vi "Plotmatrix Appearance Page.vi"() -> ()   [LabVIEW 2020, in "XY Plot Matrix.lvclass"]
uses:
  <vilib>/Math Plots/2D Math Plots/XY Plot Matrix/XY Plot Matrix/XY Plot Matrix.lvclass
  <vilib>/Math Plots/2D Math Plots/2D Plot/2D Plot/Typedef/Graph General Property.ctl
  <vilib>/Math Plots/2D Math Plots/2D Plot/Action String/XYPlotMatrix Ctrl Act Queue.ctl
  <vilib>/Math Plots/2D Math Plots/2D Plot/Action String/XYPlotMatrix Ctrl Act Cluster.ctl
  <vilib>/Math Plots/2D Math Plots/2D Plot/Action String/2DMathPlot State Class.ctl
  <vilib>/Math Plots/2D Math Plots/2D Plot/2D Plot/Typedef/Dialog State.ctl
  <vilib>/Math Plots/2D Math Plots/2D Plot/2D Plot/Typedef/Temp Graph Property Action.ctl
  <vilib>/Math Plots/2D Math Plots/2D Plot/2D Plot/Typedef/Temp Graph State.ctl
  <vilib>/Math Plots/2D Math Plots/2D Plot/2D Plot/2D Plot.lvclass
panel:
  in  "Event Registration":refnum<event-registration>
  in  "Control Ref Queue":T1
  out "Graph General Out":T2
  in  "Graph General In":T2
  in  "Legend:Plots Shown":u32=1 caption="Plots shown" min=1
  in  "Autosize Legend":bool caption="Auto size to plot names"
  in  "Legend:Visible":bool caption="Show plot legend"
  in  "Palette:Visible":bool caption="Show graph palette"
  in  "Height":u32 step=1
  in  "Width":u32 step=1
  in  "Enabled State":T3(radio)
  in  "Caption.Visible":bool caption="Caption"
  in  "Caption.Text":string caption="Caption Text"
  in  "Label.Text":string caption="Label Text"
  in  "Label.Visible":bool caption="Label"
  # "Caption"
  # "Label"
  # "Enabled State"
  # "Size"
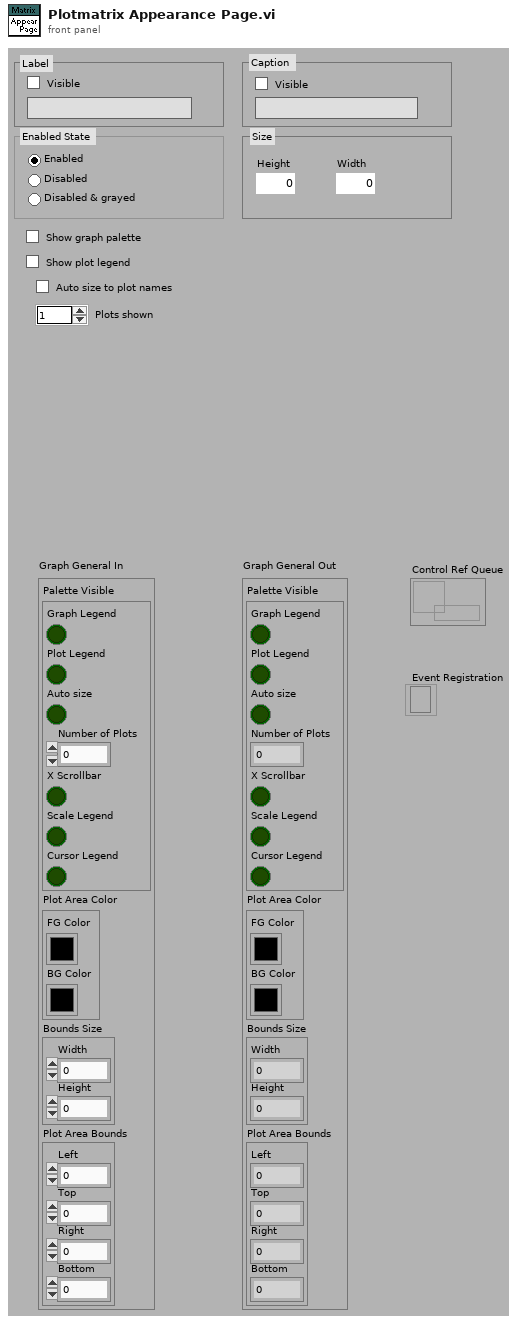
[diagram p1: front panel]
types:
  T1 = typedef "XYPlotMatrix Ctrl Act Queue.ctl" = refnum<queue>
  T2 = typedef "2D Plot.lvclass/Graph General Property.ctl" = cluster{"Palette Visible":cluster{"Graph Legend":bool, "Plot Legend":bool, "Auto size":bool, "Number of Plots":u32, "X Scrollbar":bool, "Scale Legend":bool, "Cursor Legend":bool}, "Plot Area Color":cluster{"FG Color":u32, "BG Color":u32}, "Bounds Size":cluster{"Width":u32, "Height":u32}, "Plot Area Bounds":cluster{"Left":i16, "Top":i16, "Right":i16, "Bottom":i16}}
  T3 = enum32{"Enabled", "Disabled", "Disabled & grayed", "Multiple Values"}
  T4 = typedef "2D Plot.lvclass/Dialog State.ctl" = enum16{"Initialize", "Read Property", "Write Property", "Idle", "Exit"}
  T5 = typedef "XYPlotMatrix Ctrl Act Cluster.ctl" = cluster{"Facade VI":refnum<vi>, "XControl":refnum<vi>, "Sub Panel":refnum<vi>, "Sub VI":refnum<vi>, "Export Image":refnum<vi>, "Display State Change Class":T6}
  T6 = typedef "2DMathPlot State Class.ctl" = enum16{"Update All (Undo)", "Update General", "Update Appearance", "Update Format", "Update Scale", "Update Marker", "Update Cursor", "None"}
  T7 = typedef "2D Plot.lvclass/Temp Graph State.ctl" = enum16{"Create", "Update Graph", "Update Property Only", "Get Plot Name", "Get Axis Name", "Destory"}
  T8 = typedef "2D Plot.lvclass/Temp Graph Property Action.ctl" = enum16{"Appearance Property", "Format Property", "Plots Property", "Scales Property"}
  T9 = enum8{"Enabled", "Disabled", "Disabled and Grayed Out"}
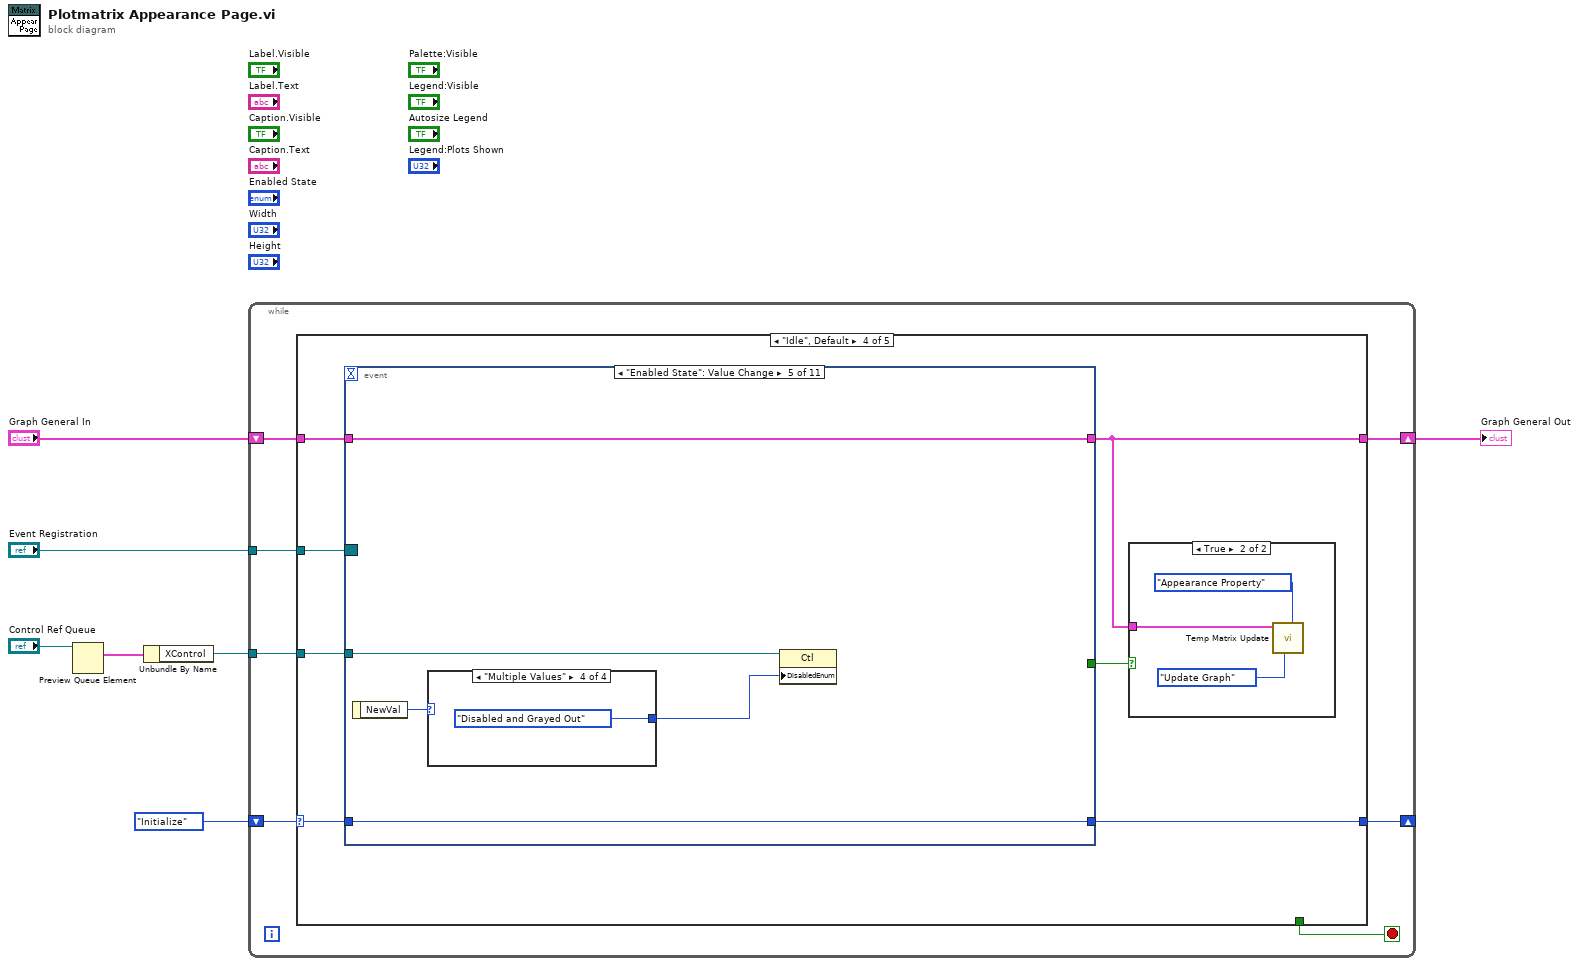
[diagram p0: block diagram]
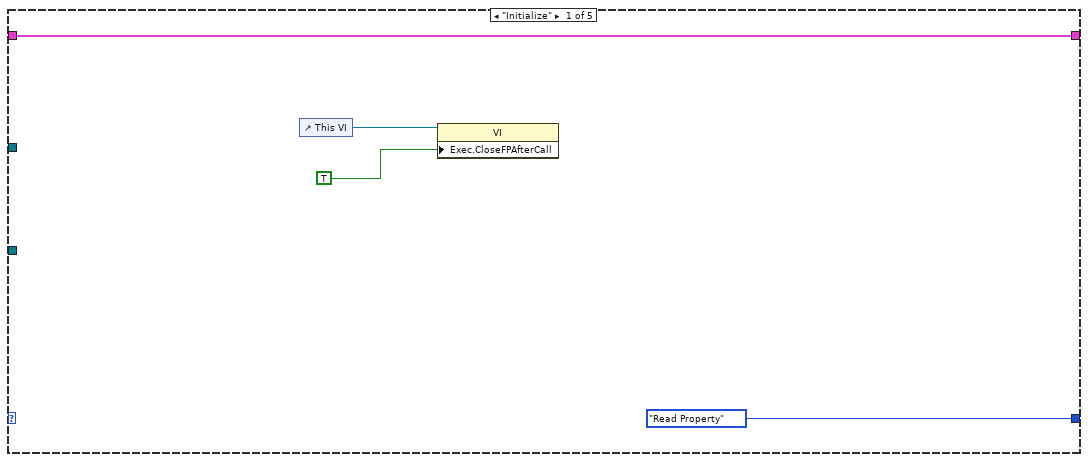
[diagram p2: hidden frame]
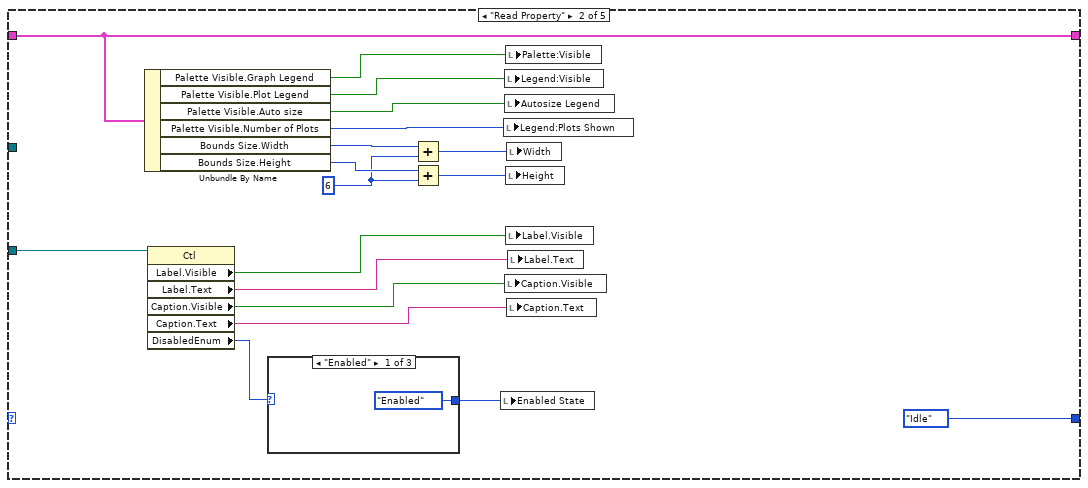
[diagram p3: hidden frame]
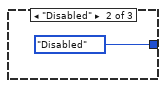
[diagram p4: hidden frame]
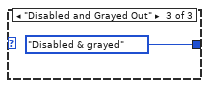
[diagram p5: hidden frame]
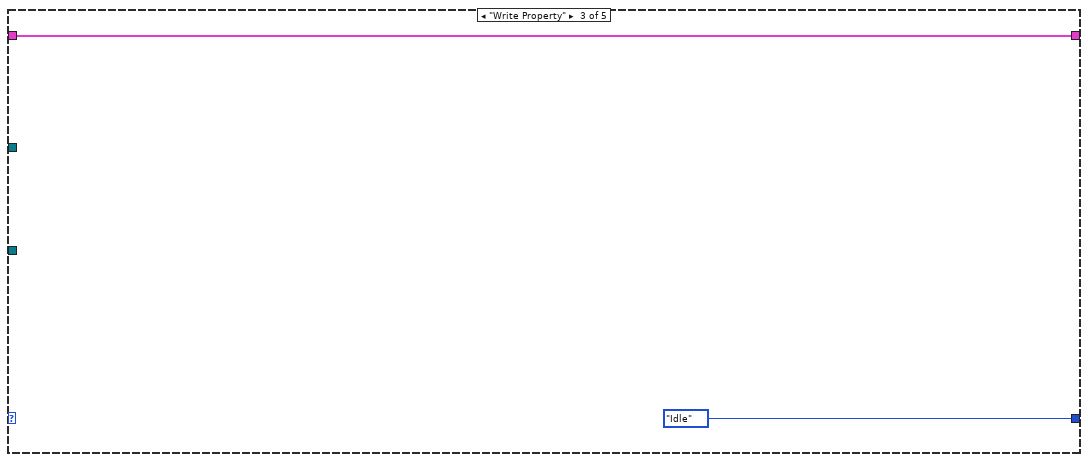
[diagram p6: hidden frame]
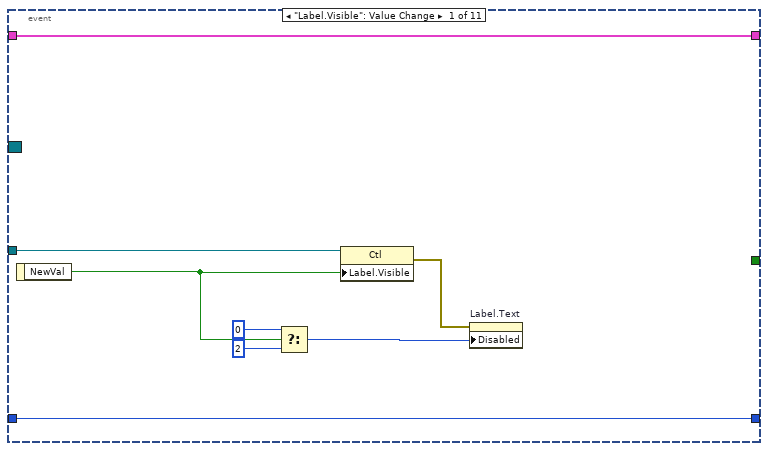
[diagram p8: hidden frame]
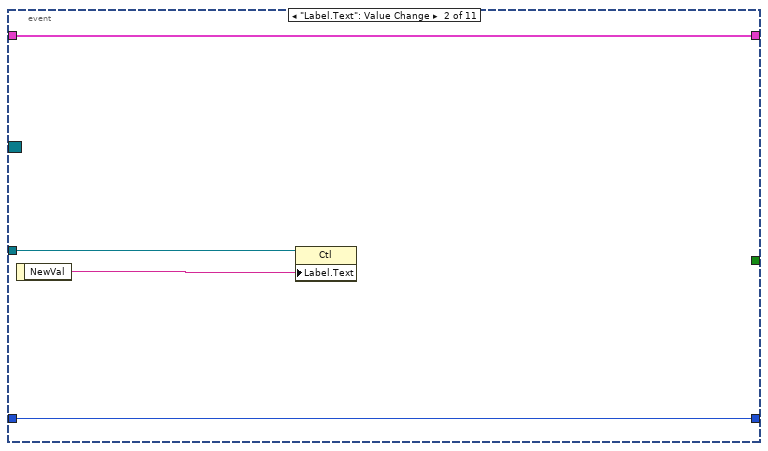
[diagram p9: hidden frame]
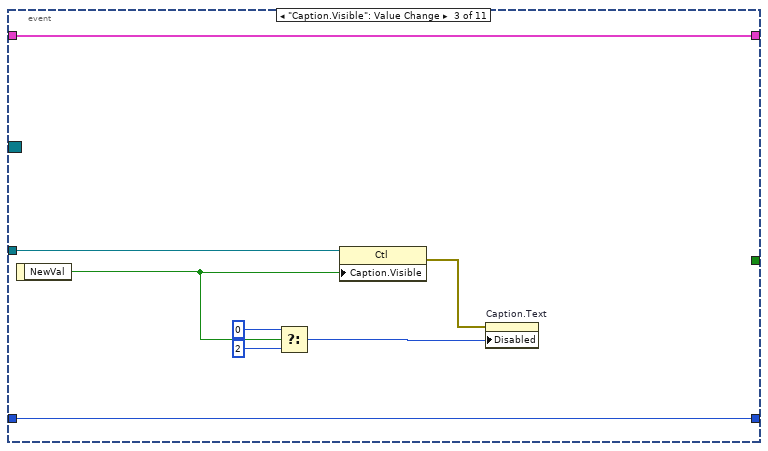
[diagram p10: hidden frame]
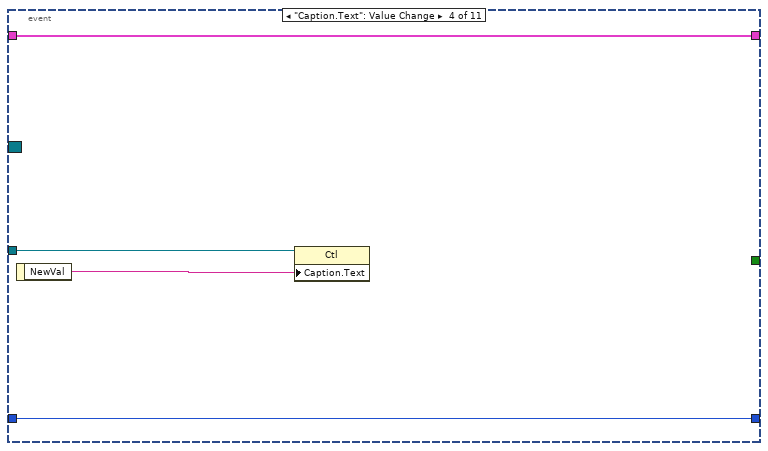
[diagram p11: hidden frame]
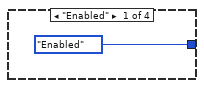
[diagram p12: hidden frame]
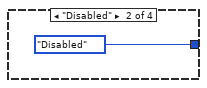
[diagram p13: hidden frame]
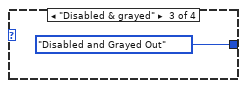
[diagram p14: hidden frame]
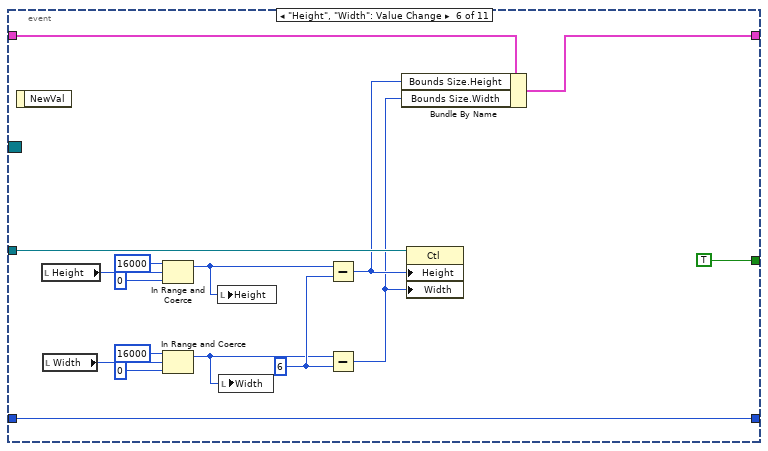
[diagram p15: hidden frame]
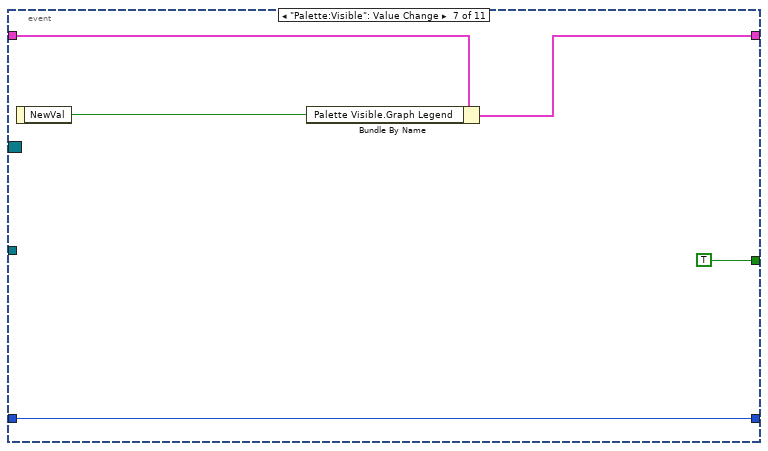
[diagram p16: hidden frame]
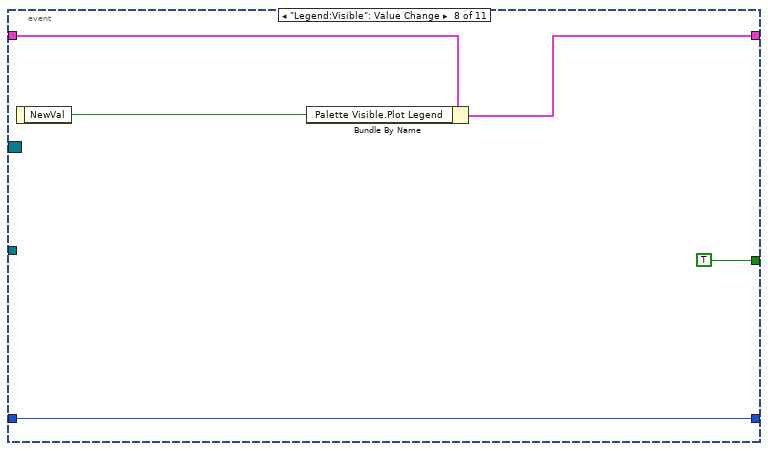
[diagram p17: hidden frame]
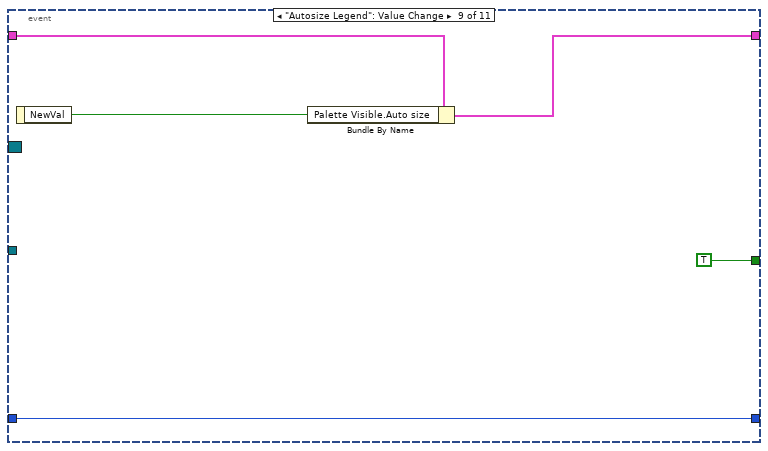
[diagram p18: hidden frame]
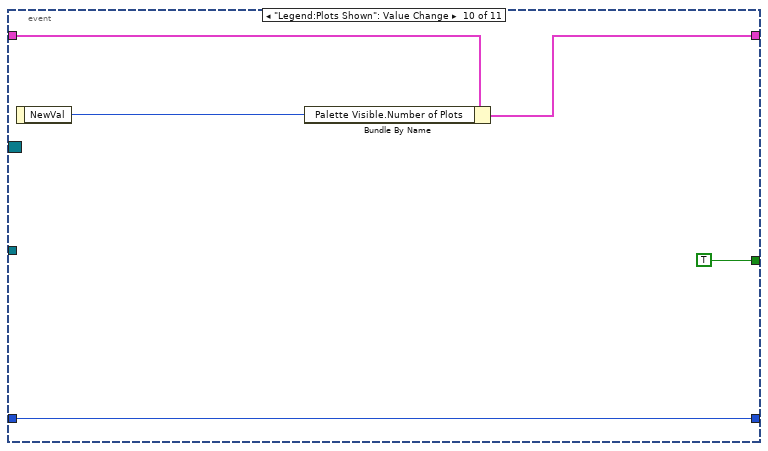
[diagram p19: hidden frame]
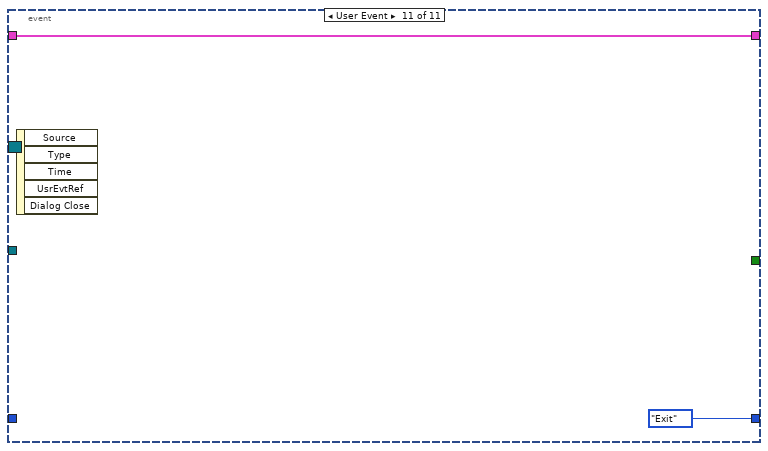
[diagram p20: hidden frame]
diagram:
  n1 = Preview Queue Element(queue="Control Ref Queue") -> (element=w1:T5)  [unwired: 1 in, 4 out]
  n2 = Unbundle By Name(w1) -> ("XControl"=w3:refnum<vi>)
  n3 = while {
    shift-right: [w12] -> _
    shift-left: Dialog_State."Initialize" ("Enum") -> [w14]
    shift-right: [w11] -> w6
    shift-left: "Graph General In" -> [w10]
    tunnel: w3 -> [w9]
    tunnel: "Event Registration" -> [w8]
    stop <- w13 stop-if-true
    n4 = case shown="\"Idle\", Default" w14 {
      selector: w14 -> [_ _ _ w44 w124]
      tunnel: [_ _ _ _ TRUE] -> w13
      tunnel: [Dialog_State."Read Property" ("Enum") Dialog_State."Idle" ("Enum") Dialog_State."Idle" ("Enum") w45 w124] -> w12
      tunnel: [w15 w26 w40 w42 w123] -> w11
      tunnel: w10 -> [w15 w26 w40 w48 w123]
      tunnel: w9 -> [_ w31 _ w47 _]
      tunnel: w8 -> [_ _ _ w46 _]
      frame "Initialize" {
        n5 = control-ref of="This VI"() -> (w17:refnum<vi>)
        n6 = property class="VI"(reference=w17, "Exec.CloseFPAfterCall"=TRUE ("Execution:Close After Call")) -> ()  [unwired: 1 in, 2 out]
      }
      frame "Read Property" {
        w21 = u32 6 ("y")
        n7 = Unbundle By Name(w26) -> ("Palette Visible.Graph Legend"=w35:bool, "Palette Visible.Plot Legend"=w34:bool, "Palette Visible.Auto size"=w33:bool, "Palette Visible.Number of Plots"=w32:u32, "Bounds Size.Width"=w25:u32, "Bounds Size.Height"=w24:u32)
        n8 = property class="Ctl"(reference=w31) -> ("Label.Visible"=w30:bool, "Label.Text"=w29:string, "Caption.Visible"=w28:bool, "Caption.Text"=w27:string, "DisabledEnum"=w20:T9)  [unwired: 1 in, 2 out]
        n9 = case shown="\"Enabled\"" w20 {
          tunnel: [T3."Enabled" ("Enabled State") T3."Disabled" ("Enabled State") T3."Disabled & grayed" ("Enabled State")] -> w19
          frame "Enabled" {
          }
          frame "Disabled" {
          }
          frame "Disabled and Grayed Out" {
          }
        }
        n10 = Add(x=w25, y=w21) -> (x+y=w23:u32)
        n11 = Add(x=w24, y=w21) -> (x+y=w22:u32)
        n12 = local write "Enabled State"(w19) -> ()
        n13 = local write "Legend:Plots Shown"(w32) -> ()
        n14 = local write "Legend:Visible"(w34) -> ()
        n15 = local write "Autosize Legend"(w33) -> ()
        n16 = local write "Caption.Visible"(w28) -> ()
        n17 = local write "Palette:Visible"(w35) -> ()
        n18 = local write "Height"(w22) -> ()
        n19 = local write "Label.Visible"(w30) -> ()
        n20 = local write "Width"(w23) -> ()
        n21 = local write "Caption.Text"(w27) -> ()
        n22 = local write "Label.Text"(w29) -> ()
      }
      frame "Write Property" {
      }
      frame "Idle", Default {
        n23 = event shown="[4] \"Enabled State\": Value Change" {
          selector: w46 -> [_ _ _ _ _ _ _ _ _ _ _]
          dyn-events: _ -> [_ _ _ _ _ _ _ _ _ _ _]
          timeout: _ -> [_ _ _ _ _ _ _ _ _ _ _]
          tunnel: w48 -> [w59 w61 w71 w73 w79 w100 w105 w110 w115 w120 w122]
          tunnel: [w59 w61 w71 w73 w79 w98 w104 w109 w114 w119 w122] -> w42
          tunnel: w47 -> [w58 w63 w70 w75 w80 w96 _ _ _ _ _]
          tunnel: [w52 w60 w64 w72 w78 w99 w102 w107 w112 w117 Dialog_State."Exit" ("Enum")] -> w45
          tunnel: w44 -> [w52 w60 w64 w72 w78 w99 w102 w107 w112 w117 _]
          tunnel: [_ _ _ _ _ TRUE TRUE TRUE TRUE TRUE _] -> w43
          event "Label.Visible": Value Change {
            n24 = event-data() -> ("NewVal"=w57:bool)  [unwired: 1 out]
            n25 = Select(t=u8 0 ("Disabled"), s=w57, f=u8 2 ("Disabled")) -> (s? t:f=w54:u8)
            n26 = property class="Ctl"(reference=w58, "Label.Visible"=w57) -> (error out=w53:errorcluster)  [unwired: 1 in, 1 out]
            n27 = property on="Label.Text" class="Str"(error in=w53, "Disabled"=w54) -> ()  [unwired: 1 in, 2 out]
          }
          event "Label.Text": Value Change {
            n28 = event-data() -> ("NewVal"=w62:string)  [unwired: 1 out]
            n29 = property class="Ctl"(reference=w63, "Label.Text"=w62) -> ()  [unwired: 1 in, 2 out]
          }
          event "Caption.Visible": Value Change {
            n30 = event-data() -> ("NewVal"=w69:bool)  [unwired: 1 out]
            n31 = Select(t=u8 0 ("Disabled"), s=w69, f=u8 2 ("Disabled")) -> (s? t:f=w66:u8)
            n32 = property class="Ctl"(reference=w70, "Caption.Visible"=w69) -> (error out=w65:errorcluster)  [unwired: 1 in, 1 out]
            n33 = property on="Caption.Text" class="Str"(error in=w65, "Disabled"=w66) -> ()  [unwired: 1 in, 2 out]
          }
          event "Caption.Text": Value Change {
            n34 = event-data() -> ("NewVal"=w74:string)  [unwired: 1 out]
            n35 = property class="Ctl"(reference=w75, "Caption.Text"=w74) -> ()  [unwired: 1 in, 2 out]
          }
          event "Enabled State": Value Change {
            n36 = event-data() -> ("NewVal"=w77:T3)  [unwired: 1 out]
            n37 = case shown="\"Multiple Values\"" w77 {
              tunnel: [T9."Enabled" ("Disabled") T9."Disabled" ("Disabled") T9."Disabled and Grayed Out" ("Disabled") T9."Disabled and Grayed Out" ("Disabled")] -> w76
              frame "Enabled" {
              }
              frame "Disabled" {
              }
              frame "Disabled & grayed" {
              }
              frame "Multiple Values" {
              }
            }
            n38 = property class="Ctl"(reference=w80, "DisabledEnum"=w76) -> ()  [unwired: 1 in, 2 out]
          }
          event "Height", "Width": Value Change {
            w93 = u32 6 ("x")
            n39 = event-data() -> ()  [unwired: 2 out]
            n40 = local read "Height"() -> (w88:u32)
            n41 = local read "Width"() -> (w87:u32)
            n42 = In Range and Coerce(upper limit=u32 16000, x=w88, lower limit=u32 0) -> (coerced(x)=w85:u32)  [unwired: 1 out]
            n43 = In Range and Coerce(upper limit=u32 16000, x=w87, lower limit=u32 0) -> (coerced(x)=w86:u32)  [unwired: 1 out]
            n44 = local write "Height"(w85) -> ()
            n45 = local write "Width"(w86) -> ()
            n46 = Subtract(x=w85, y=w93) -> (x-y=w95:u32)
            n47 = Subtract(x=w86, y=w93) -> (x-y=w94:u32)
            n48 = Bundle By Name(cluster=w100, "Bounds Size.Height"=w95, "Bounds Size.Width"=w94) -> (w98:T2)
            n49 = property class="Ctl"(reference=w96, "Height"=w95, "Width"=w94) -> ()  [unwired: 1 in, 2 out]
          }
          event "Palette:Visible": Value Change {
            n50 = event-data() -> ("NewVal"=w103:bool)  [unwired: 1 out]
            n51 = Bundle By Name(cluster=w105, "Palette Visible.Graph Legend"=w103) -> (w104:T2)
          }
          event "Legend:Visible": Value Change {
            n52 = event-data() -> ("NewVal"=w108:bool)  [unwired: 1 out]
            n53 = Bundle By Name(cluster=w110, "Palette Visible.Plot Legend"=w108) -> (w109:T2)
          }
          event "Autosize Legend": Value Change {
            n54 = event-data() -> ("NewVal"=w113:bool)  [unwired: 1 out]
            n55 = Bundle By Name(cluster=w115, "Palette Visible.Auto size"=w113) -> (w114:T2)
          }
          event "Legend:Plots Shown": Value Change {
            n56 = event-data() -> ("NewVal"=w118:u32)  [unwired: 1 out]
            n57 = Bundle By Name(cluster=w120, "Palette Visible.Number of Plots"=w118) -> (w119:T2)
          }
          event User Event {
            n58 = event-data() -> ()  [unwired: 6 out]
          }
        }
        n59 = case shown="True" w43 {
          tunnel: w42 -> [_ w51]
          frame False {
          }
          frame True {
            n60 = call <vilib>:"Temp Matrix Update.vi"("Property Name"=Temp_Graph_Property_Action."Appearance Property", "State"=Temp_Graph_State."Update Graph", "Property In"=w51) -> ()  [unwired: 2 in, 7 out]
          }
        }
      }
      frame "Exit" {
      }
    }
  }
  "Graph General Out" <- w6
